vi "FL_Get_Histogram_Bin_value.vi"(1 "Current value":dbl format="%#_13g", 2 "Bins array":dbl[](array[numeric])) -> (0 "Bin assignment":i32)   [LabVIEW 2018, in "Tracker.lvlib"]
uses:
  Tracker.lvlib
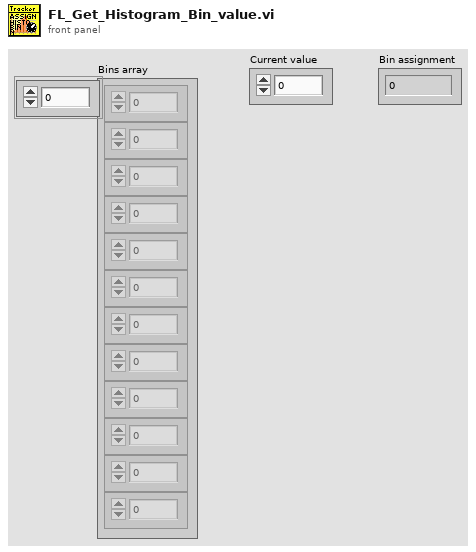
[diagram p1: front panel]
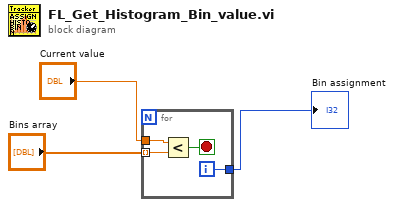
[diagram p0: block diagram]
diagram:
  n1 = for {
    tunnel: "Bins array" -> [w6] mode=indexing
    tunnel: "Current value" -> [w7]
    tunnel: [w4] -> w1
    i -> [w4]
    stop <- w5 stop-if-true
    n2 = Less?(x=w7, y=w6) -> (x < y?=w5:bool)
  }
  "Bin assignment" <- w1
